vi "StarTrekIndicator.vi"(2 "Counter":i32) -> (7 "Back and Forth":bool[](array[boolean]), 9 "Forward":bool[](array[boolean]))   [LabVIEW 2016]
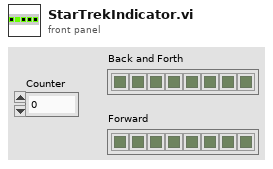
[diagram p1: front panel]
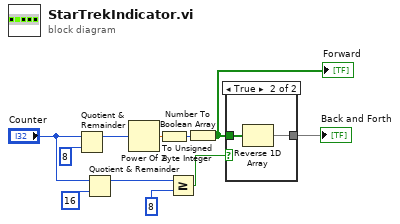
[diagram p0: block diagram]
diagram:
  n1 = Quotient & Remainder(x="Counter", y=8 ("x")) -> (x-y*floor(x/y)=w11:i32)  [unwired: 1 out]
  n2 = Quotient & Remainder(x="Counter", y=16 ("x")) -> (x-y*floor(x/y)=w5:i32)  [unwired: 1 out]
  n3 = Power Of 2(x=w11) -> (2^x=w9:dbl)
  n4 = To Unsigned Byte Integer(number=w9) -> (unsigned 8bit integer=w8:u8)
  n5 = Greater Or Equal?(x=w5, y=8 ("x")) -> (x >= y?=w3:bool)
  n6 = Number To Boolean Array(number=w8) -> (Boolean array=w1:bool[])
  "Forward" <- w1
  n7 = case shown="True" w3 {
    tunnel: w1 -> [w12 w14]
    tunnel: [w12 w13] -> w2
    frame False {
    }
    frame True {
      n8 = Reverse 1D Array(array=w14) -> (reversed array=w13:bool[])
    }
  }
  "Back and Forth" <- w2
